vi "Compare Timestamps.vi"(1 "Unit (ms)":T1=enum."millisecond", 2 "timestamp (1)":timestamp, 3 "timestamp (2)":timestamp, 4 "Resolution (in selected unit)":dbl=1.0) -> (7 "Equal?":bool)   [LabVIEW 2018]
doc: "Timestamp is not converted to UTC time, so the year being evaluated is the year of the timestamp, not the current year at GMT."
uses:
  <vilib>/LabVIEW Open Source Project/Epoch Date & Time/Timestamp Compare Units -- enum.ctl
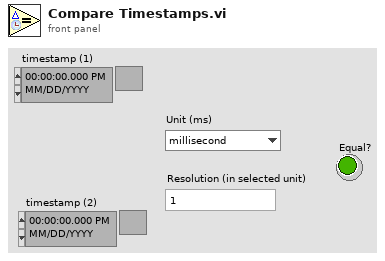
[diagram p1: front panel]
types:
  T1 = typedef "Timestamp Compare Units -- enum.ctl" = enum16{"week", "day", "hour", "minute", "second", "millisecond", "microsecond", "nanosecond"}
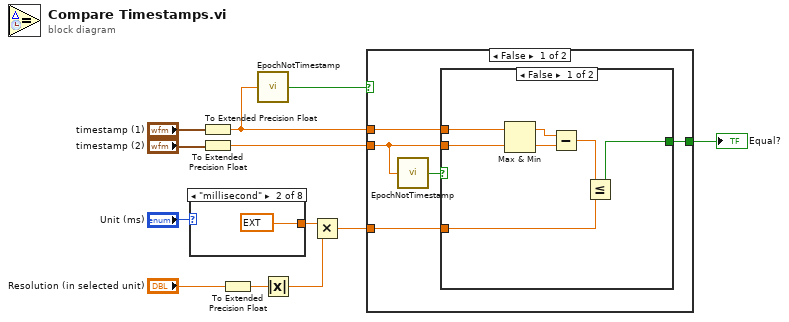
[diagram p0: block diagram]
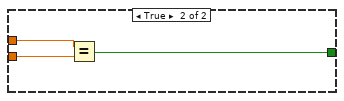
[diagram p3: hidden frame]
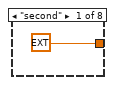
[diagram p4: hidden frame]
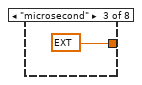
[diagram p5: hidden frame]
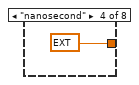
[diagram p6: hidden frame]
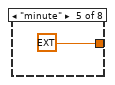
[diagram p7: hidden frame]
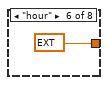
[diagram p8: hidden frame]
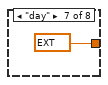
[diagram p9: hidden frame]
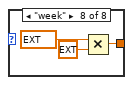
[diagram p10: hidden frame]
diagram:
  n1 = case shown="\"millisecond\"" "Unit (ms)" {
    tunnel: [ext 1.0 ext 0.00099999999999999999996 ext 0.00000100000000000000000004 ext 1e-9 ext 60.0 ext 3600.0 ext 86400.0 w20] -> w10
    frame "second" {
    }
    frame "millisecond" {
    }
    frame "microsecond" {
    }
    frame "nanosecond" {
    }
    frame "minute" {
    }
    frame "hour" {
    }
    frame "day" {
    }
    frame "week" {
      n2 = Multiply(x=ext 86400.0, y=ext 7.0) -> (x*y=w20:ext)
    }
  }
  n3 = To Extended Precision Float(1:"timestamp (1)") -> (0:w5:ext)
  n4 = To Extended Precision Float(1:"timestamp (2)") -> (0:w6:ext)
  n5 = To Extended Precision Float(1:"Resolution (in selected unit)") -> (0:w2:ext)
  n6 = call <vilib>:"EpochNotTimestamp.vi"("Epoch Time"=w5) -> ("Not a Timestamp?"=w4:bool)  [unwired: 8 in]
  n7 = Absolute Value(x=w2) -> (abs(x)=w9:ext)
  n8 = Multiply(x=w10, y=w9) -> (x*y=w3:ext)
  n9 = case shown="False" w4 {
    tunnel: w6 -> [w26 w37]
    tunnel: w5 -> [w27 w36]
    tunnel: w3 -> [w24 _]
    tunnel: [w23 w35] -> w1
    frame False {
      n10 = call <vilib>:"EpochNotTimestamp.vi"("Epoch Time"=w26) -> ("Not a Timestamp?"=w25:bool)  [unwired: 8 in]
      n11 = case shown="False" w25 {
        tunnel: w26 -> [w34 _]
        tunnel: w27 -> [w31 _]
        tunnel: w24 -> [w29 _]
        tunnel: [w28 _] -> w23
        frame False {
          n12 = Max & Min(x=w31, y=w34) -> (max(x,y)=w32:ext, min(x,y)=w33:ext)
          n13 = Subtract(x=w32, y=w33) -> (x-y=w30:ext)
          n14 = Less Or Equal?(x=w30, y=w29) -> (x <= y?=w28:bool)
        }
        frame True {
        }
      }
    }
    frame True {
      n15 = Equal?(x=w36, y=w37) -> (x = y?=w35:bool)
    }
  }
  "Equal?" <- w1
